vi "uTTA_ReadCAL_File.vi"(8 "error in":errorcluster, 11 "file path":path) -> (0 "error out":errorcluster, 1 "ADC":cluster{"Offset":dbl[], "Gain":dbl[]}, 2 "PGA":cluster{"Offset":dbl[], "Gain":dbl[]})   [LabVIEW 2021]
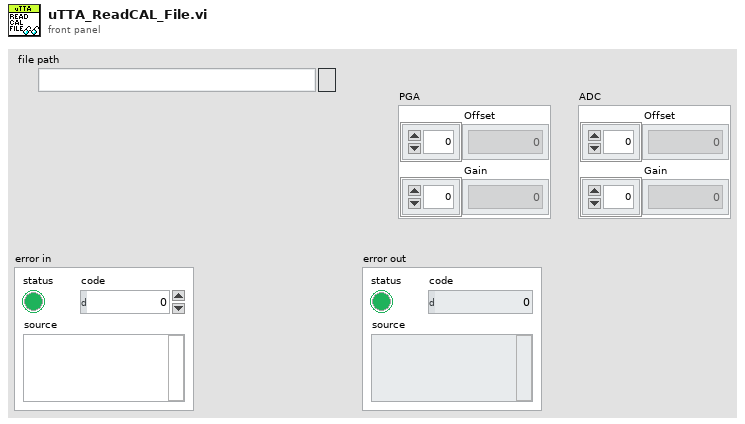
[diagram p1: front panel]
types:
  T1 = enum16{"open", "open or create", "create or replace", "create", "open (read-only)"}
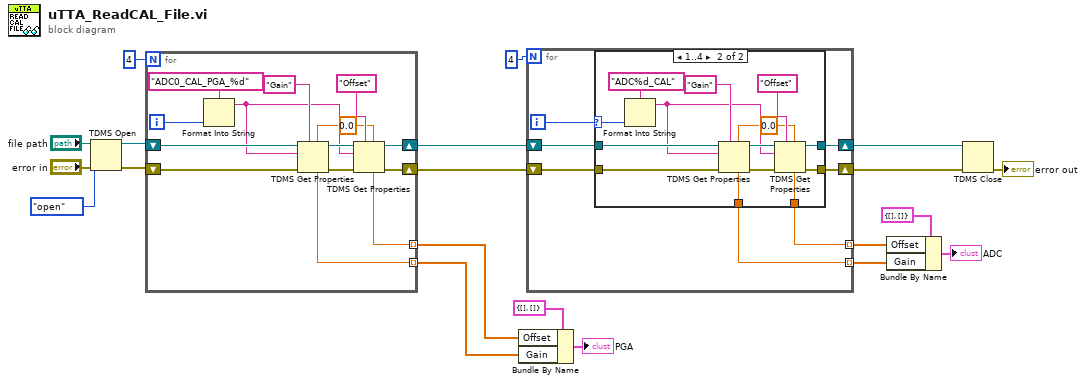
[diagram p0: block diagram]
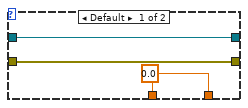
[diagram p2: hidden frame]
diagram:
  n1 = TDMS Open(8:"error in", 10:T1."open" ("operation (0:open)"), 11:"file path") -> (0:w20:errorcluster, 3:w19:refnum<k34>)  [unwired: 4 in]
  n2 = for {
    N: 4 -> [_]
    shift-right: [w26] -> w12
    shift-left: w19 -> [w34]
    shift-right: [w25] -> w11
    shift-left: w20 -> [w33]
    tunnel: [w23] -> w5 mode=indexing
    tunnel: [w22] -> w6 mode=indexing
    i -> [w21]
    w24 = 0.0
    n3 = Format Into String(format string="ADC0_CAL_PGA_%d", w21) -> (resulting string=w28:string)  [unwired: 2 in, 1 out]
    n4 = TDMS Get Properties(5:w24, 7:"Gain", 8:w33, 10:w28, 11:w34) -> (0:w30:errorcluster, 3:w29:refnum<k34>, 4:w23:dbl)  [unwired: 1 in, 3 out]
    n5 = TDMS Get Properties(5:w24, 7:"Offset", 8:w30, 10:w28, 11:w29) -> (0:w25:errorcluster, 3:w26:refnum<k34>, 4:w22:dbl)  [unwired: 1 in, 3 out]
  }
  n6 = Bundle By Name(cluster=cluster{"Offset":dbl[], "Gain":dbl[]} {"Offset"=[], "Gain"=[]} ("input cluster"), "Offset"=w6, "Gain"=w5) -> (→"PGA":cluster{"Offset":dbl[], "Gain":dbl[]})
  n7 = for {
    N: 4 -> [_]
    shift-right: [w39] -> w10
    shift-left: w12 -> [w41]
    shift-right: [w38] -> w9
    shift-left: w11 -> [w40]
    tunnel: [w37] -> w2 mode=indexing
    tunnel: [w36] -> w3 mode=indexing
    i -> [w35]
    n8 = case shown="1..4" w35 {
      selector: w35 -> [_ w45]
      tunnel: w41 -> [w44 w58]
      tunnel: w40 -> [w43 w57]
      tunnel: [w44 w50] -> w39
      tunnel: [w43 w49] -> w38
      tunnel: [w42 w47] -> w37
      tunnel: [w42 w46] -> w36
      frame Default {
        w42 = 0.0
      }
      frame 1..4 {
        w48 = 0.0
        n9 = Format Into String(format string="ADC%d_CAL", w45) -> (resulting string=w52:string)  [unwired: 2 in, 1 out]
        n10 = TDMS Get Properties(5:w48, 7:"Gain", 8:w57, 10:w52, 11:w58) -> (0:w54:errorcluster, 3:w53:refnum<k34>, 4:w47:dbl)  [unwired: 1 in, 3 out]
        n11 = TDMS Get Properties(5:w48, 7:"Offset", 8:w54, 10:w52, 11:w53) -> (0:w49:errorcluster, 3:w50:refnum<k34>, 4:w46:dbl)  [unwired: 1 in, 3 out]
      }
    }
  }
  n12 = Bundle By Name(cluster=cluster{"Offset":dbl[], "Gain":dbl[]} {"Offset"=[], "Gain"=[]} ("input cluster"), "Offset"=w3, "Gain"=w2) -> (→"ADC":cluster{"Offset":dbl[], "Gain":dbl[]})
  n13 = TDMS Close(8:w9, 11:w10) -> (0:→"error out":errorcluster)  [unwired: 1 out]
